vi "AFPP Pre-Install Custom Action.vi"(10 "Variant":variant) -> (0 "error out":errorcluster)   [LabVIEW 2020]
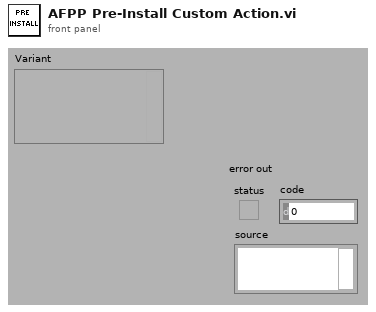
[diagram p1: front panel]
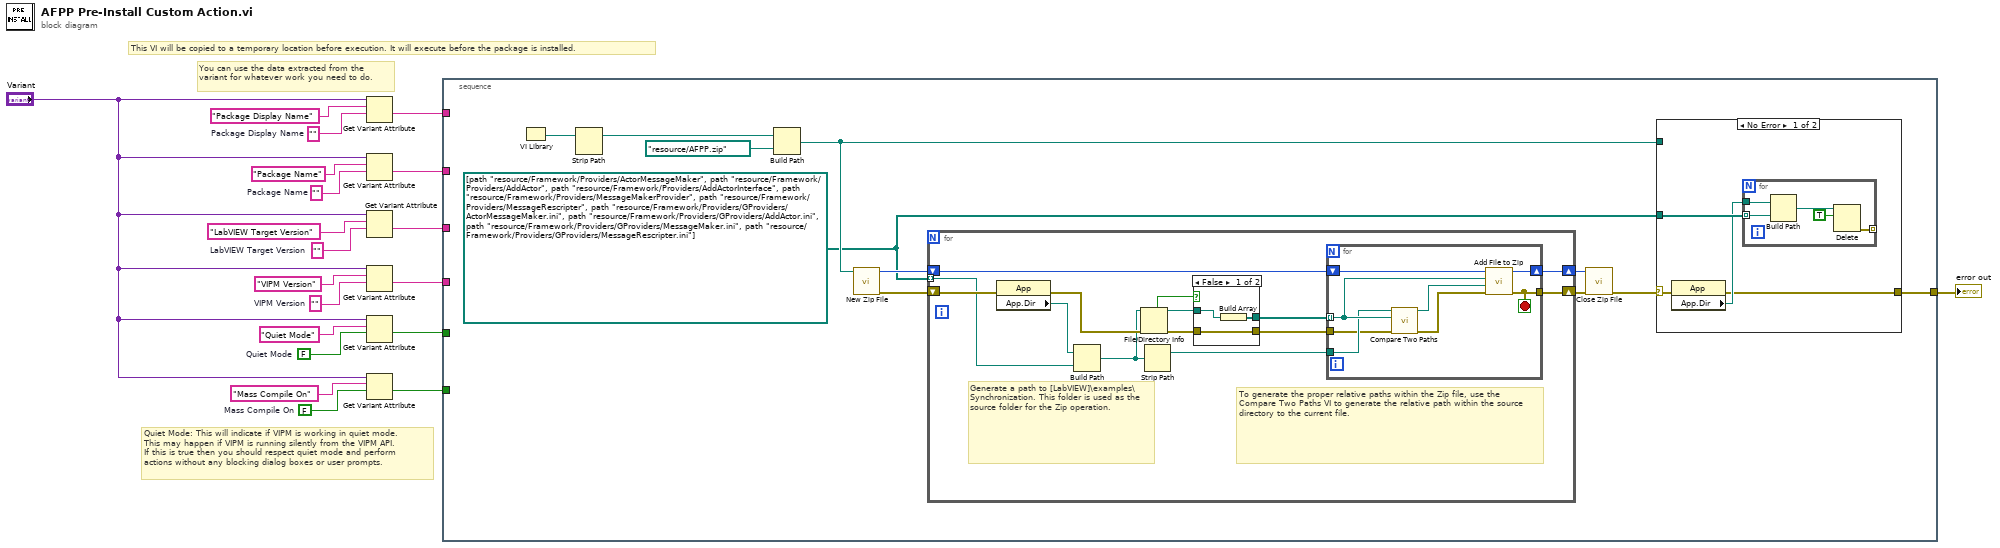
[diagram p0: block diagram]
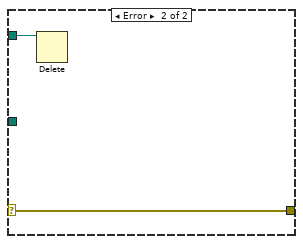
[diagram p2: hidden frame]
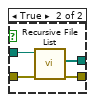
[diagram p3: hidden frame]
diagram:
  w2 = FALSE  # Mass Compile On
  w4 = ""  # Package Display Name
  w11 = FALSE  # Quiet Mode
  w14 = ""  # VIPM Version
  w16 = ""  # LabVIEW Target Version
  w18 = ""  # Package Name
  # "You can use the data extracted from the variant for whatever work you need to do."
  # "Quiet Mode: This will indicate if VIPM is working in quiet mode.\nThis may happen if VIPM is running silently from the VIPM API.\nIf this is true then you should respect quiet mode and perform\nactions without any blocking dialog boxes or user prompts."
  # "This VI will be copied to a temporary location before execution. It will execute before the package is installed."
  n1 = Get Variant Attribute(Variant="Variant", name="Package Display Name", default value (empty Variant)=w4) -> (value=w10:string)  [unwired: 1 in, 3 out]
  n2 = Get Variant Attribute(Variant="Variant", name="Package Name", default value (empty Variant)=w18) -> (value=w9:string)  [unwired: 1 in, 3 out]
  n3 = Get Variant Attribute(Variant="Variant", name="LabVIEW Target Version", default value (empty Variant)=w16) -> (value=w8:string)  [unwired: 1 in, 3 out]
  n4 = Get Variant Attribute(Variant="Variant", name="VIPM Version", default value (empty Variant)=w14) -> (value=w7:string)  [unwired: 1 in, 3 out]
  n5 = Get Variant Attribute(Variant="Variant", name="Quiet Mode", default value (empty Variant)=w11) -> (value=w6:bool)  [unwired: 1 in, 3 out]
  n6 = Get Variant Attribute(Variant="Variant", name="Mass Compile On", default value (empty Variant)=w2) -> (value=w5:bool)  [unwired: 1 in, 3 out]
  n7 = stacked-sequence {
    tunnel: w10 -> [_]
    tunnel: w9 -> [_]
    tunnel: w8 -> [_]
    tunnel: w7 -> [_]
    tunnel: w6 -> [_]
    tunnel: w5 -> [_]
    tunnel: [w31] -> w1
    frame #0 {
      w22 = path[] [path "resource/Framework/Providers/ActorMessageMaker", path "resource/Framework/Providers/AddActor", path "resource/Framework/Providers/AddActorInterface", path "resource/Framework/Providers/MessageMakerProvider", path "resource/Framework/Providers/MessageRescripter", path "resource/Framework/Providers/GProviders/ActorMessageMaker.ini", path "resource/Framework/Providers/GProviders/AddActor.ini", path "resource/Framework/Providers/GProviders/MessageMaker.ini", path "resource/Framework/Providers/GProviders/MessageRescripter.ini"]
      n8 = VI Library() -> (path=w24:path)
      n9 = Strip Path(path=w24) -> (stripped path=w21:path)  [unwired: 1 out]
      n10 = Build Path(base path=w21, name or relative path=path "resource/AFPP.zip") -> (appended path=w30:path)
      n11 = call <vilib>:"New Zip File.vi"("target"=w30) -> ("error out"=w26:errorcluster, "zip file out"=w25:i64)  [unwired: 2 in, 3 out]
      n12 = for {
        shift-right: [w55] -> w27
        shift-left: w26 -> [w56]
        tunnel: w22 -> [w54] mode=indexing
        shift-right: [w43] -> w28
        shift-left: w25 -> [w53]
        # "Generate a path to [LabVIEW]\\examples\\Synchronization. This folder is used as the source folder for the Zip operation."
        # "To generate the proper relative paths within the Zip file, use the Compare Two Paths VI to generate the relative path within the source directory to the current file."
        n13 = property class="App"(error in=w56) -> (error out=w52:errorcluster, "App.Dir"=w45:path)  [unwired: 1 in, 1 out]
        n14 = Build Path(base path=w45, name or relative path=w54) -> (appended path=w48:path)
        n15 = File/Directory Info(path=w48, error in=w52) -> (path out=w49:path, directory=w50:bool, error out=w47:errorcluster)  [unwired: 4 out]
        n16 = Strip Path(path=w48) -> (stripped path=w51:path)  [unwired: 1 out]
        n17 = case shown="False" w50 {
          tunnel: [w57 w63] -> w44
          tunnel: [w59 w62] -> w46
          tunnel: w47 -> [w59 w61]
          tunnel: w49 -> [w58 w60]
          frame False {
            n18 = Build Array(w58) -> (w57:path[])
          }
          frame True {
            n19 = call <vilib>:"Recursive File List.vi"("error in (no error)"=w61, "Folder Path"=w60) -> ("error out"=w62:errorcluster, "All Files in Dir"=w63:path[])  [unwired: 5 in, 3 out]
          }
        }
        n20 = for {
          tunnel: w44 -> [w68] mode=indexing
          tunnel: w46 -> [w65]
          tunnel: [w69] -> w55
          shift-right: [w70] -> w43
          shift-left: w53 -> [w71]
          tunnel: w51 -> [w67]
          stop <- w69 stop-if-true
          n21 = call <vilib>:"Compare Two Paths.vi"("error in (no error)"=w65, "Path 2"=w68, "Path 1"=w67) -> ("error out"=w64:errorcluster, "Relative Path from 1 to 2"=w66:path)  [unwired: 5 in, 2 out]
          n22 = call <vilib>:"Add File to Zip.vi"("error in (no error)"=w64, "destination path in zip"=w66, "source file path"=w68, "zip file in"=w71) -> ("error out"=w69:errorcluster, "zip file out"=w70:i64)  [unwired: 6 out]
        }
      }
      n23 = call <vilib>:"Close Zip File.vi"("error in (no error)"=w27, "zip file in"=w28) -> ("error out"=w29:errorcluster)  [unwired: 1 in, 4 out]
      n24 = case shown="No Error" w29 {
        selector: w29 -> [w35 w42]
        tunnel: [w32 w42] -> w31
        tunnel: w30 -> [_ w41]
        tunnel: w22 -> [w34 _]
        frame No Error {
          n25 = property class="App"(error in=w35) -> (error out=w32:errorcluster, "App.Dir"=w33:path)  [unwired: 1 in, 1 out]
          n26 = for {
            tunnel: w34 -> [w40] mode=indexing
            tunnel: w33 -> [w38]
            tunnel: [w37] -> _ mode=indexing
            n27 = Build Path(base path=w38, name or relative path=w40) -> (appended path=w39:path)
            n28 = Delete(path (use dialog)=w39, entire hierarchy (F)=TRUE) -> (error out=w37:errorcluster)  [unwired: 3 in, 2 out]
          }
        }
        frame Error {
          n29 = Delete(path (use dialog)=w41) -> ()  [unwired: 4 in, 3 out]
        }
      }
    }
  }
  "error out" <- w1
